vi "Creat_Traj_Config_Convert_V5_To_V_internal.vi"(11 "TrajCreateConfig V5":T5={"Write Config File Name"=path "", "Write Config File Comment"="", "WayPoints"=[], "TRAJECTORY_CONFIG_V4"={"MaxVelocity"=0.0, "Max Acceleration"=0.0, "StartVelocity"=0.0, "End Velocity"=0.0, "Reversed"=FALSE, "DiffDrKineConstntDefined"=FALSE, "CentAcellConstntDefined"=FALSE, "DiffDrVoltConstntDefined"=FALSE, "DIFF_DRIVE_KINE_CONSTRAINT"={"Max Speed (M/S)"=0.0, "DIFF_DRIVE_KINEMATICS"={"TrackWidth_Meters"=0.0}, "Max Accel (M/S2)"=99999.0}, "CENTRIPETAL_ACCEL_CONSTRAINT"={"Max Cent Accel"=0.0}, "SwerveDrKineConstntDefined"=FALSE, "SWERVE_DRIVE_KINE_CONSTRAINT"={"Max Speed (M/S)"=0.0, "SwerveKinematics"={"NumModules"=0, "InverseKinematics"=[], "ForwardKinematics"=[], "Modules"=[], "PrevCoR"={"X"=0.0, "Y"=0.0}, "SavedModuleStates"=[]}}, "DIFF_DRIVE_VOLTAGE_CONSTRAINT"={"Max Voltage"=0.0, "DIFF_DRIVE_KINEMATICS"={"TrackWidth_Meters"=0.0}, "SIMPLE_MOTOR_FF"={"Ks"=0.0, "Kv"=0.0, "Ka"=0.0, "KnInv"=0.0}}, "MECANUM_DRIVE_KINE_CONSTRAINT"={"Max Speed (M/S)"=0.0, "MECA_DRIVE_KINEMATICS"={"FrontLeft"={"X"=0.0, "Y"=0.0}, "FrontRight"={"X"=0.0, "Y"=0.0}, "RearLeft"={"X"=0.0, "Y"=0.0}, "RearRight"={"X"=0.0, "Y"=0.0}, "InverseKinematics"=[[0.0, 1.0, -1.0, 0.0], [0.0, 1.0, 1.0, 0.0], [0.0, 1.0, 1.0, 0.0], [0.0, 1.0, -1.0, 0.0]], "ForwardKinematics"=[[0.0, 1.0, -1.0, 0.0], [0.0, 1.0, 1.0, 0.0], [0.0, 1.0, 1.0, 0.0], [0.0, 1.0, -1.0, 0.0]], "PrevCoR"={"X"=0.0, "Y"=0.0}}}, "MecanumDrKineConstntDefined"=FALSE}, "IsCubic"=FALSE, "Units Selector"=enum."Inches", "UseWeights"=FALSE, "FieldName"="", "Rect Region Exists"=FALSE, "RectRegionBotLeft"={"X"=0.0, "Y"=0.0}, "RectRegionTopRight"={"X"=0.0, "Y"=0.0}, "Rect Region Max Speed"=0.0} {"RectRegionTopRight"."Y" format="%14.3f"; "RectRegionTopRight"."X" format="%14.3f"; "RectRegionBotLeft"."Y" format="%14.3f"; "RectRegionBotLeft"."X" format="%14.3f"; "WayPoints"."WEIGHT" format="%13.3f"; "WayPoints"."ANGLE" format="%13.3f"; "WayPoints"."Y" format="%13.3f"; "WayPoints"."X" format="%13.3f"; "TRAJECTORY_CONFIG_V4"."MECANUM_DRIVE_KINE_CONSTRAINT"."MECA_DRIVE_KINEMATICS"."PrevCoR"."Y" format="%14.3f"; "TRAJECTORY_CONFIG_V4"."MECANUM_DRIVE_KINE_CONSTRAINT"."MECA_DRIVE_KINEMATICS"."PrevCoR"."X" format="%14.3f"; "TRAJECTORY_CONFIG_V4"."MECANUM_DRIVE_KINE_CONSTRAINT"."MECA_DRIVE_KINEMATICS"."RearRight"."Y" format="%14.3f"; "TRAJECTORY_CONFIG_V4"."MECANUM_DRIVE_KINE_CONSTRAINT"."MECA_DRIVE_KINEMATICS"."RearRight"."X" format="%14.3f"; "TRAJECTORY_CONFIG_V4"."MECANUM_DRIVE_KINE_CONSTRAINT"."MECA_DRIVE_KINEMATICS"."RearLeft"."Y" format="%14.3f"; "TRAJECTORY_CONFIG_V4"."MECANUM_DRIVE_KINE_CONSTRAINT"."MECA_DRIVE_KINEMATICS"."RearLeft"."X" format="%14.3f"; "TRAJECTORY_CONFIG_V4"."MECANUM_DRIVE_KINE_CONSTRAINT"."MECA_DRIVE_KINEMATICS"."FrontRight"."Y" format="%14.3f"; "TRAJECTORY_CONFIG_V4"."MECANUM_DRIVE_KINE_CONSTRAINT"."MECA_DRIVE_KINEMATICS"."FrontRight"."X" format="%14.3f"; "TRAJECTORY_CONFIG_V4"."MECANUM_DRIVE_KINE_CONSTRAINT"."MECA_DRIVE_KINEMATICS"."FrontLeft"."Y" format="%14.3f"; "TRAJECTORY_CONFIG_V4"."MECANUM_DRIVE_KINE_CONSTRAINT"."MECA_DRIVE_KINEMATICS"."FrontLeft"."X" format="%14.3f"; "TRAJECTORY_CONFIG_V4"."MECANUM_DRIVE_KINE_CONSTRAINT"."Max Speed (M/S)" format="%20.4f"; "TRAJECTORY_CONFIG_V4"."DIFF_DRIVE_VOLTAGE_CONSTRAINT"."SIMPLE_MOTOR_FF"."KnInv" format="%13.4f"; "TRAJECTORY_CONFIG_V4"."DIFF_DRIVE_VOLTAGE_CONSTRAINT"."SIMPLE_MOTOR_FF"."Ka" format="%13.4f"; "TRAJECTORY_CONFIG_V4"."DIFF_DRIVE_VOLTAGE_CONSTRAINT"."SIMPLE_MOTOR_FF"."Kv" format="%13.4f"; "TRAJECTORY_CONFIG_V4"."DIFF_DRIVE_VOLTAGE_CONSTRAINT"."SIMPLE_MOTOR_FF"."Ks" format="%13.4f"; "TRAJECTORY_CONFIG_V4"."DIFF_DRIVE_VOLTAGE_CONSTRAINT"."DIFF_DRIVE_KINEMATICS"."TrackWidth_Meters" format="%20.4f"; "TRAJECTORY_CONFIG_V4"."DIFF_DRIVE_VOLTAGE_CONSTRAINT"."Max Voltage" format="%20.4f"; "TRAJECTORY_CONFIG_V4"."SWERVE_DRIVE_KINE_CONSTRAINT"."SwerveKinematics"."PrevCoR"."Y" format="%14.3f"; "TRAJECTORY_CONFIG_V4"."SWERVE_DRIVE_KINE_CONSTRAINT"."SwerveKinematics"."PrevCoR"."X" format="%14.3f"; "TRAJECTORY_CONFIG_V4"."SWERVE_DRIVE_KINE_CONSTRAINT"."SwerveKinematics"."Modules"."Y" format="%14.3f"; "TRAJECTORY_CONFIG_V4"."SWERVE_DRIVE_KINE_CONSTRAINT"."SwerveKinematics"."Modules"."X" format="%14.3f"; "TRAJECTORY_CONFIG_V4"."SWERVE_DRIVE_KINE_CONSTRAINT"."Max Speed (M/S)" format="%20.4f"; "TRAJECTORY_CONFIG_V4"."CENTRIPETAL_ACCEL_CONSTRAINT"."Max Cent Accel" format="%20.4f"; "TRAJECTORY_CONFIG_V4"."DIFF_DRIVE_KINE_CONSTRAINT"."Max Accel (M/S2)" format="%20.4f"; "TRAJECTORY_CONFIG_V4"."DIFF_DRIVE_KINE_CONSTRAINT"."DIFF_DRIVE_KINEMATICS"."TrackWidth_Meters" format="%20.4f"; "TRAJECTORY_CONFIG_V4"."DIFF_DRIVE_KINE_CONSTRAINT"."Max Speed (M/S)" format="%20.4f"; "TRAJECTORY_CONFIG_V4"."End Velocity" format="%20.4f"; "TRAJECTORY_CONFIG_V4"."StartVelocity" format="%20.4f"; "TRAJECTORY_CONFIG_V4"."Max Acceleration" format="%20.4f"; "TRAJECTORY_CONFIG_V4"."MaxVelocity" format="%20.4f"}) -> (3 "TrajCreateConfig V_Internal":T1 {"WayPoints"."WEIGHT" format="%13.3f"; "WayPoints"."ANGLE" format="%13.3f"; "WayPoints"."Y" format="%13.3f"; "WayPoints"."X" format="%13.3f"; "TRAJECTORY_CONFIG"."End Velocity" format="%20.4f"; "TRAJECTORY_CONFIG"."StartVelocity" format="%20.4f"; "TRAJECTORY_CONFIG"."Max Acceleration" format="%20.4f"; "TRAJECTORY_CONFIG"."MaxVelocity" format="%20.4f"})   [LabVIEW 2019]
uses:
  CreateTrajectoryTypeDef/TrajCreateConfig_V5.ctl
  <vilib>/Rock Robotics/WPI/ThirdParty/JAS_Junk/TrajLib/TypeDef/DISPLAY_WEIGHTED_WAYPOINT.ctl
  CreateTrajectoryTypeDef/TrajCreateTrajConfig_V4.ctl
  <vilib>/Rock Robotics/WPI/ThirdParty/JAS_Junk/TrajLib/TypeDef/TRAJ_CONSTRAINT_DIIF_DRIVE_KINEMATICS.ctl
  <vilib>/Rock Robotics/WPI/ThirdParty/JAS_Junk/TrajLib/TypeDef/DIFF_DRIVE_KINEMATICS.ctl
  <vilib>/Rock Robotics/WPI/ThirdParty/JAS_Junk/TrajLib/TypeDef/TRAJ_CONSTRAINT_CENTRIPETAL_ACCEL.ctl
  <vilib>/Rock Robotics/WPI/ThirdParty/JAS_Junk/TrajLib/TypeDef/TRAJ_CONSTRAINT_SWERVE_DRIVE_KINEMATICS.ctl
  <vilib>/Rock Robotics/WPI/ThirdParty/JAS_Junk/TrajLib/TypeDef/SWERVE_DRIVE_KINEMATICS.ctl
  <vilib>/Analysis/Matrix/Datatypes/RealMatrix.ctl
  <vilib>/Rock Robotics/WPI/ThirdParty/JAS_Junk/TrajLib/TypeDef/TRANSLATION2D.ctl
  <vilib>/Rock Robotics/WPI/ThirdParty/JAS_Junk/TrajLib/TypeDef/SWERVE_DRIVE_MODULE_STATE.ctl
  <vilib>/Rock Robotics/WPI/ThirdParty/JAS_Junk/TrajLib/TypeDef/ROTATION2D.ctl
  <vilib>/Rock Robotics/WPI/ThirdParty/JAS_Junk/TrajLib/TypeDef/TRAJ_CONSTRAINT_DIIF_DRIVE_VOLTAGE.ctl
  <vilib>/Rock Robotics/WPI/ThirdParty/JAS_Junk/TrajLib/TypeDef/SIMPLE_MOTOR_FF.ctl
  <vilib>/Rock Robotics/WPI/ThirdParty/JAS_Junk/TrajLib/TypeDef/TRAJ_CONSTRAINT_MECA_DRIVE_KINEMATICS.ctl
  <vilib>/Rock Robotics/WPI/ThirdParty/JAS_Junk/TrajLib/TypeDef/MECA_DRIVE_KINEMATICS.ctl
  CreateTrajectoryENUM/TrajCreateUnitsENUM.ctl
  CreateTrajectoryTypeDef/TrajCreateConfig__V_Internal.ctl
  <vilib>/Rock Robotics/WPI/ThirdParty/JAS_Junk/TrajLib/TypeDef/TRAJ_CONFIG.ctl
  <vilib>/Rock Robotics/WPI/ThirdParty/JAS_Junk/TrajLib/VI/TrajConstraint_GetType.vi
  <vilib>/Utility/Data Type/Get Type Information.vi
  <vilib>/Rock Robotics/WPI/ThirdParty/JAS_Junk/TrajLib/Trajectory_Library.lvlib
  <vilib>/Analysis/Matrix/NI_Matrix.lvlib
panel:
  # "ARRAY OF OTHER\nCONSTRAINTS \nGOES HERE.."
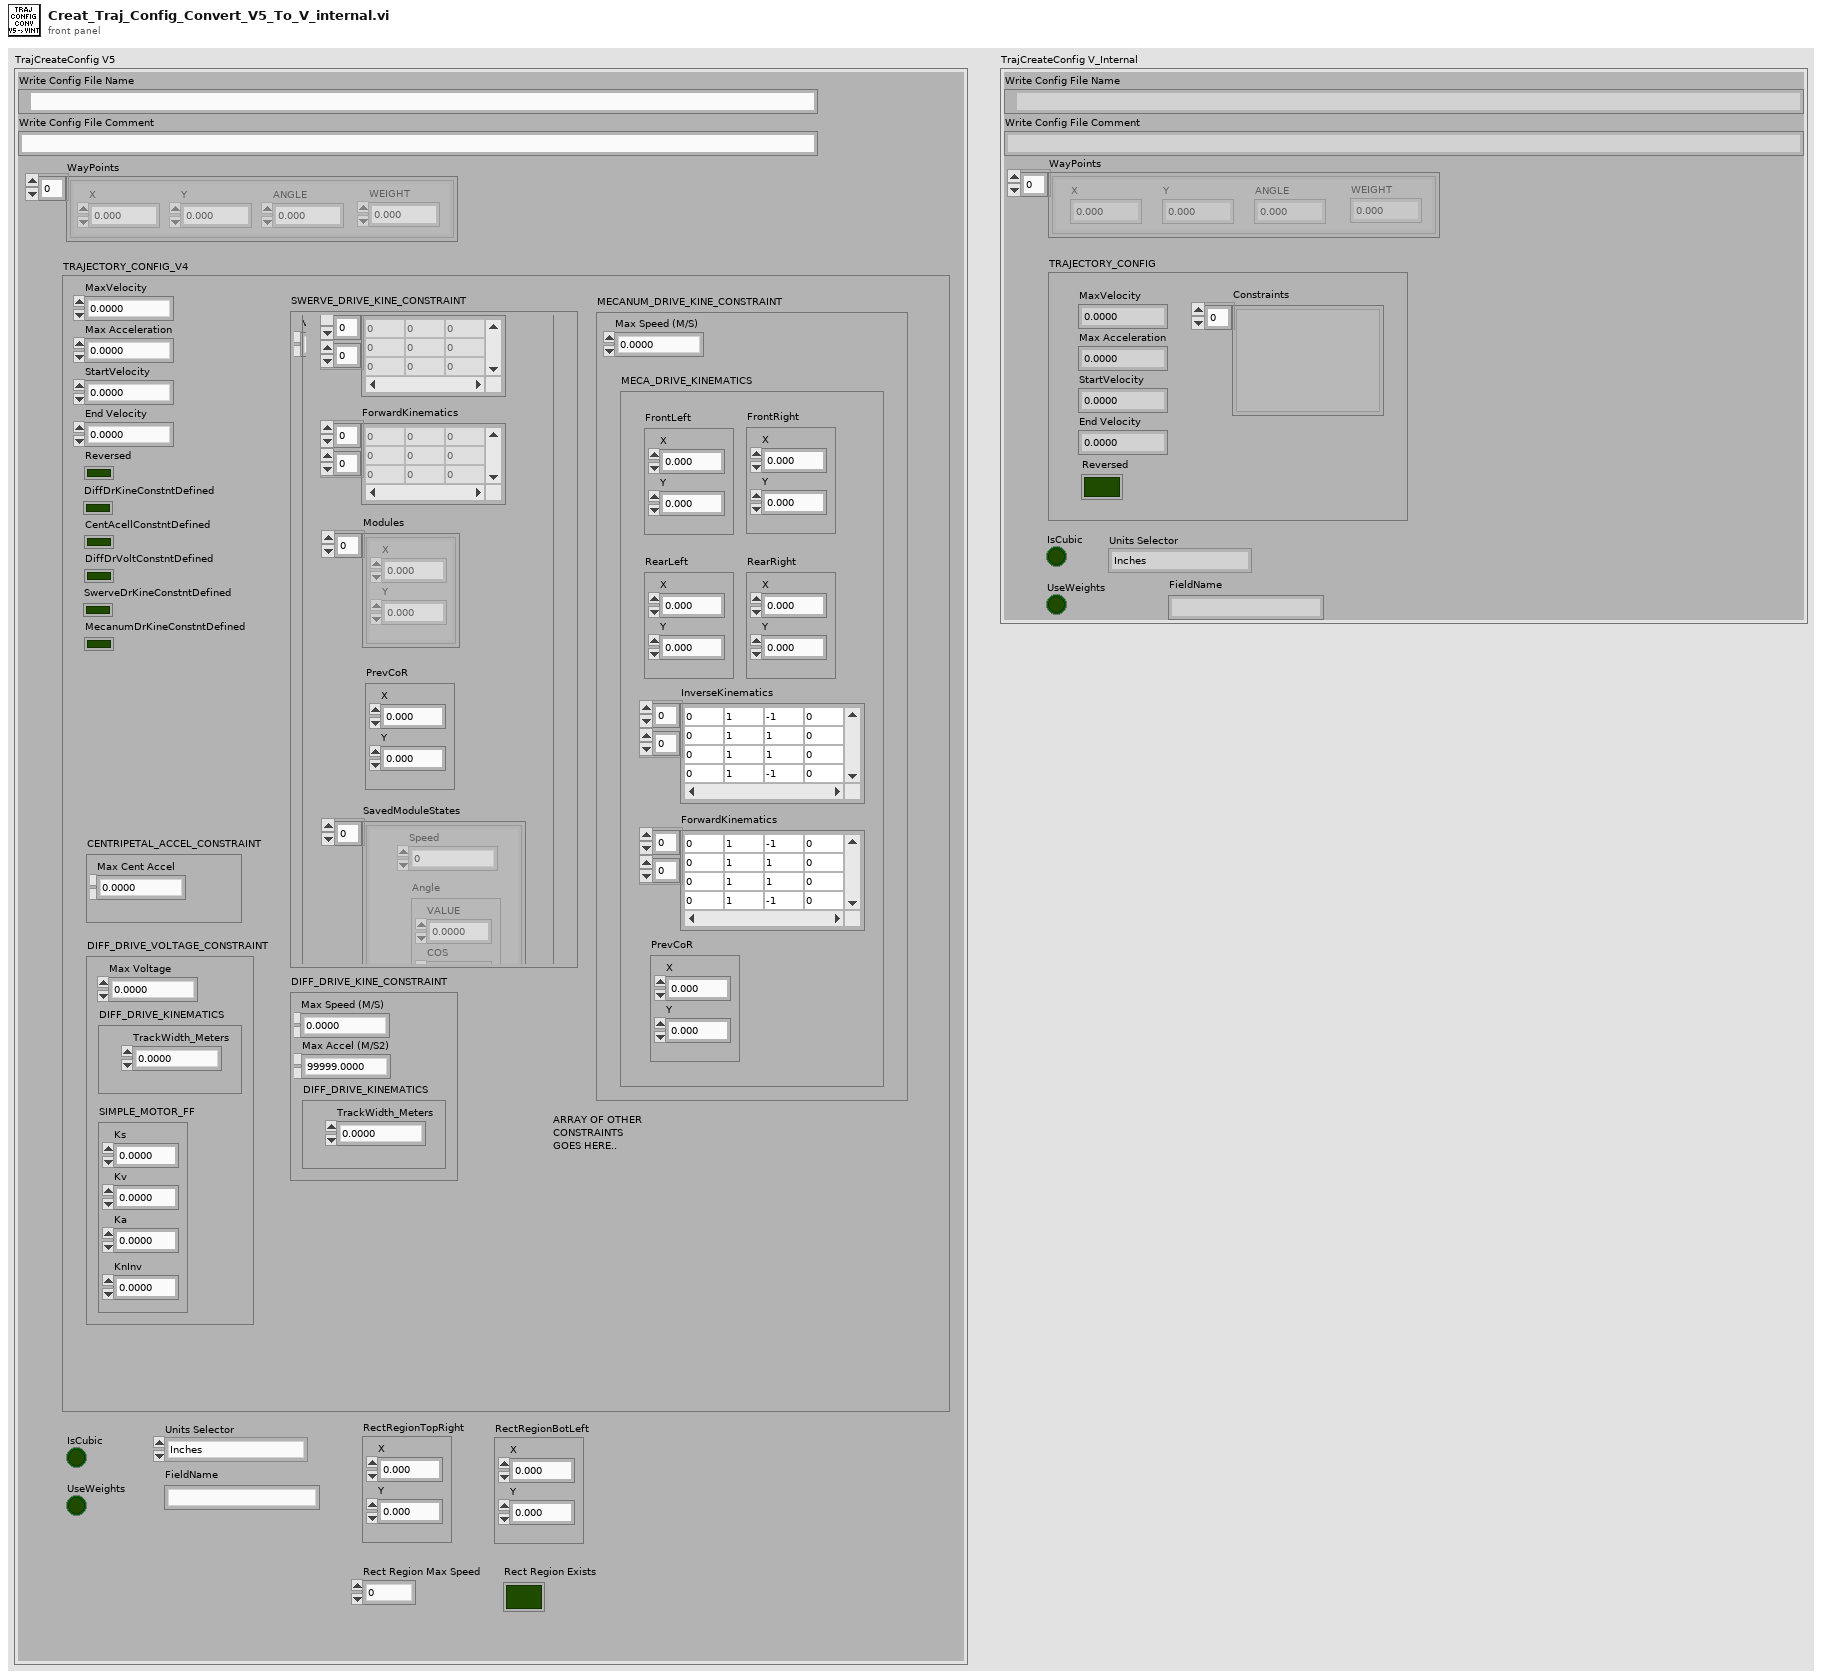
[diagram p1: front panel]
types:
  T1 = typedef "TrajCreateConfig__V_Internal.ctl" = cluster{"Write Config File Name":path, "Write Config File Comment":string, "WayPoints":T2[], "TRAJECTORY_CONFIG":T3, "IsCubic":bool, "Units Selector":T4, "UseWeights":bool, "FieldName":string}
  T2 = typedef "Trajectory_Library.lvlib/DISPLAY_WEIGHTED_WAYPOINT.ctl" = cluster{"X":dbl, "Y":dbl, "ANGLE":dbl, "WEIGHT":dbl}
  T3 = typedef "Trajectory_Library.lvlib/TRAJ_CONFIG.ctl" = cluster{"MaxVelocity":dbl, "Max Acceleration":dbl, "StartVelocity":dbl, "End Velocity":dbl, "Reversed":bool, "Constraints":variant[]}
  T4 = typedef "TrajCreateUnitsENUM.ctl" = enum16{"Inches", "Feet", "Centimeters", "Meters"}
  T5 = typedef "TrajCreateConfig_V5.ctl" = cluster{"Write Config File Name":path, "Write Config File Comment":string, "WayPoints":T2[], "TRAJECTORY_CONFIG_V4":T6, "IsCubic":bool, "Units Selector":T4, "UseWeights":bool, "FieldName":string, "Rect Region Exists":bool, "RectRegionBotLeft":T13, "RectRegionTopRight":T13, "Rect Region Max Speed":dbl}
  T6 = typedef "TrajCreateTrajConfig_V4.ctl" = cluster{"MaxVelocity":dbl, "Max Acceleration":dbl, "StartVelocity":dbl, "End Velocity":dbl, "Reversed":bool, "DiffDrKineConstntDefined":bool, "CentAcellConstntDefined":bool, "DiffDrVoltConstntDefined":bool, "DIFF_DRIVE_KINE_CONSTRAINT":T7, "CENTRIPETAL_ACCEL_CONSTRAINT":T9, "SwerveDrKineConstntDefined":bool, "SWERVE_DRIVE_KINE_CONSTRAINT":T10, "DIFF_DRIVE_VOLTAGE_CONSTRAINT":T16, "MECANUM_DRIVE_KINE_CONSTRAINT":T18, "MecanumDrKineConstntDefined":bool}
  T7 = typedef "Trajectory_Library.lvlib/TRAJ_CONSTRAINT_DIIF_DRIVE_KINEMATICS.ctl" = cluster{"Max Speed (M/S)":dbl, "DIFF_DRIVE_KINEMATICS":T8, "Max Accel (M/S2)":dbl}
  T8 = typedef "Trajectory_Library.lvlib/DIFF_DRIVE_KINEMATICS.ctl" = cluster{"TrackWidth_Meters":dbl}
  T9 = typedef "Trajectory_Library.lvlib/TRAJ_CONSTRAINT_CENTRIPETAL_ACCEL.ctl" = cluster{"Max Cent Accel":dbl}
  T10 = typedef "Trajectory_Library.lvlib/TRAJ_CONSTRAINT_SWERVE_DRIVE_KINEMATICS.ctl" = cluster{"Max Speed (M/S)":dbl, "SwerveKinematics":T11}
  T11 = typedef "Trajectory_Library.lvlib/SWERVE_DRIVE_KINEMATICS.ctl" = cluster{"NumModules":i32, "InverseKinematics":T12, "ForwardKinematics":T12, "Modules":T13[], "PrevCoR":T13, "SavedModuleStates":T14[]}
  T12 = typedef "NI_Matrix.lvlib/RealMatrix.ctl" = dbl[][]
  T13 = typedef "Trajectory_Library.lvlib/TRANSLATION2D.ctl" = cluster{"X":dbl, "Y":dbl}
  T14 = typedef "Trajectory_Library.lvlib/SWERVE_DRIVE_MODULE_STATE.ctl" = cluster{"Speed":dbl, "Angle":T15}
  T15 = typedef "Trajectory_Library.lvlib/ROTATION2D.ctl" = cluster{"VALUE":dbl, "COS":dbl, "SIN":dbl}
  T16 = typedef "Trajectory_Library.lvlib/TRAJ_CONSTRAINT_DIIF_DRIVE_VOLTAGE.ctl" = cluster{"Max Voltage":dbl, "DIFF_DRIVE_KINEMATICS":T8, "SIMPLE_MOTOR_FF":T17}
  T17 = typedef "Trajectory_Library.lvlib/SIMPLE_MOTOR_FF.ctl" = cluster{"Ks":dbl, "Kv":dbl, "Ka":dbl, "KnInv":dbl}
  T18 = typedef "Trajectory_Library.lvlib/TRAJ_CONSTRAINT_MECA_DRIVE_KINEMATICS.ctl" = cluster{"Max Speed (M/S)":dbl, "MECA_DRIVE_KINEMATICS":T19}
  T19 = typedef "Trajectory_Library.lvlib/MECA_DRIVE_KINEMATICS.ctl" = cluster{"FrontLeft":T13, "FrontRight":T13, "RearLeft":T13, "RearRight":T13, "InverseKinematics":T12, "ForwardKinematics":T12, "PrevCoR":T13}
  T20 = typedef "Trajectory_Library.lvlib/TRAJ_CONSTRAINT_MAX_VELOCITY.ctl" = cluster{"Max Velocity":dbl, "IM UNIQUE":bool}
  T21 = typedef "Trajectory_Library.lvlib/TRAJ_CONSTRAINT_RECT_REGION.ctl" = cluster{"BottomLeftPoint":T13, "TopRightPoint":T13, "Constraint":variant, "Constraint Type":T22}
  T22 = typedef "Trajectory_Library.lvlib/TRAJ_CONSTRAINT_TYPES_ENUM.ctl" = enum16{"UNDEFINED", "DIFF DRIVE KINEMATICS", "DIFF DRIVE VOLTAGE", "CENTRIPITAL ACCEL", "MECA DRIVE KINEMATICS", "SWERVE DRIVE KINEMATICS", "MAXIMUM VELOCITY", "ELLIPTICAL REGION", "RECTANGULAR REGION"}
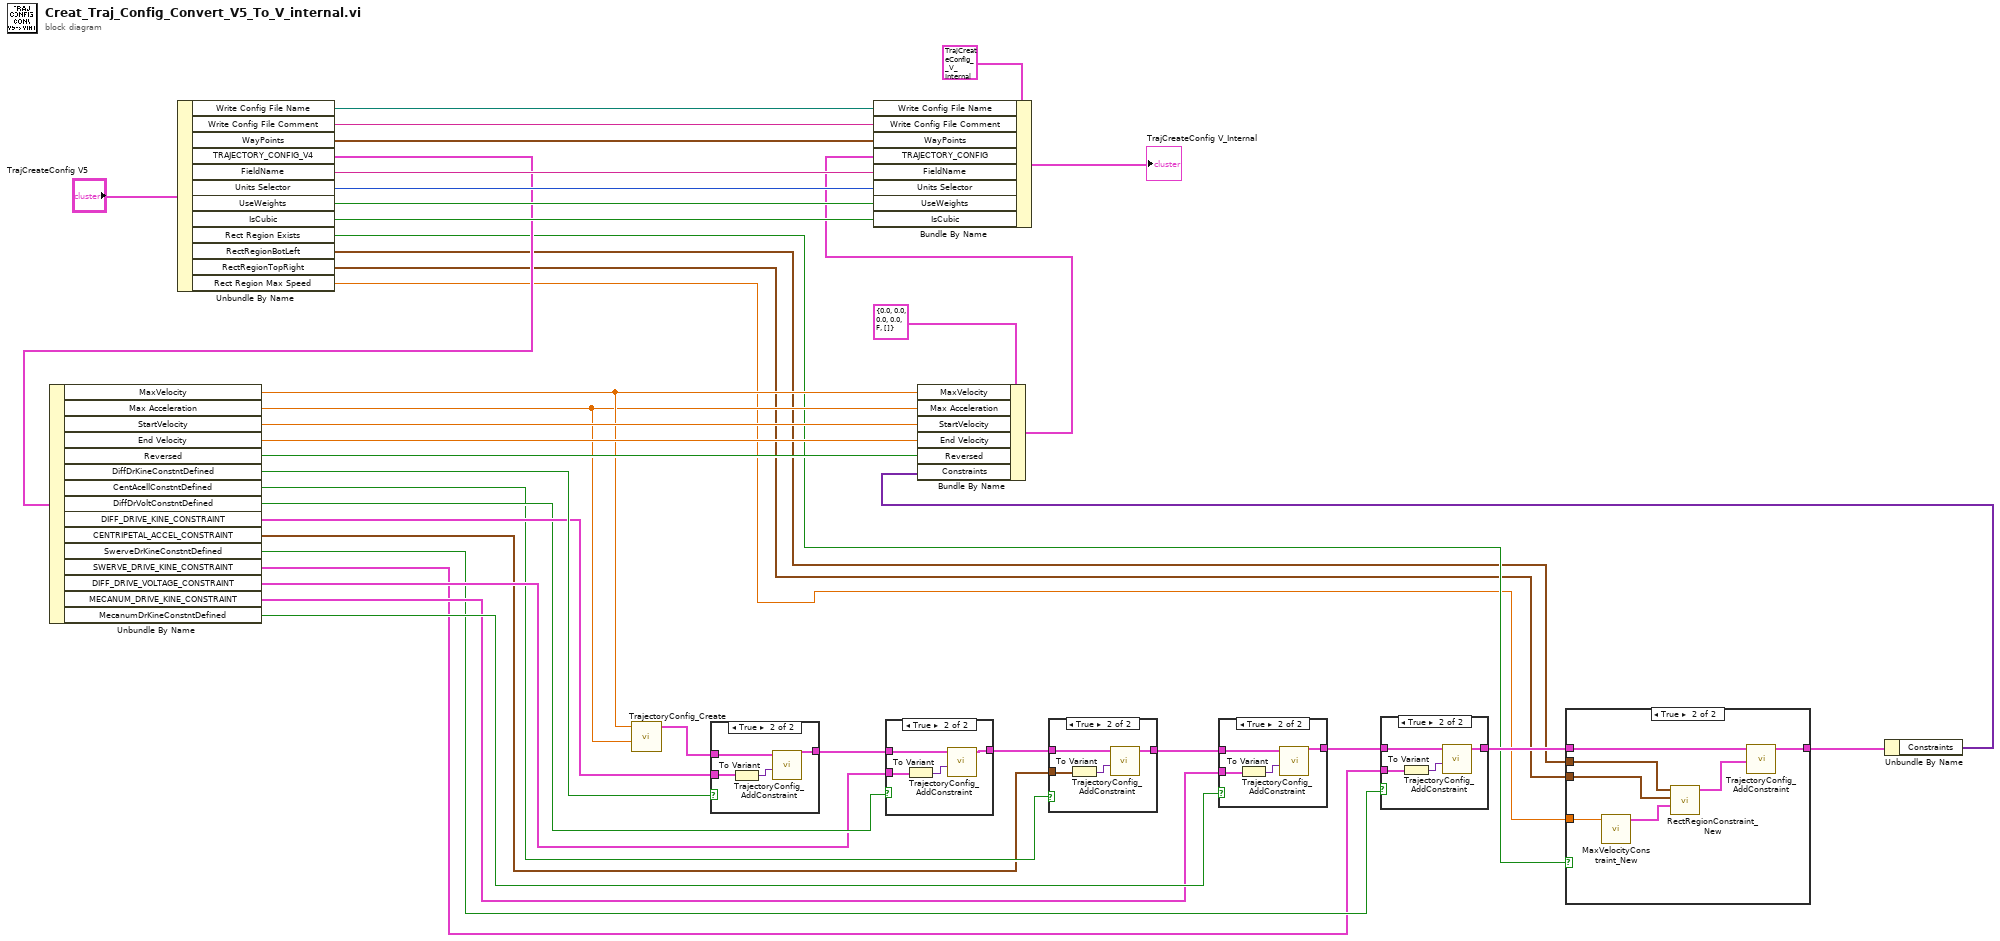
[diagram p0: block diagram]
diagram:
  n1 = Unbundle By Name("TrajCreateConfig V5") -> ("Write Config File Name"=w33:path, "Write Config File Comment"=w32:string, "WayPoints"=w31:T2[], "TRAJECTORY_CONFIG_V4"=w26:T6, "FieldName"=w30:string, "Units Selector"=w29:T4, "UseWeights"=w28:bool, "IsCubic"=w27:bool, "Rect Region Exists"=w6:bool, "RectRegionBotLeft"=w5:T13, "RectRegionTopRight"=w4:T13, "Rect Region Max Speed"=w1:dbl)
  n2 = Unbundle By Name(w26) -> ("MaxVelocity"=w21:dbl, "Max Acceleration"=w20:dbl, "StartVelocity"=w24:dbl, "End Velocity"=w23:dbl, "Reversed"=w22:bool, "DiffDrKineConstntDefined"=w18:bool, "CentAcellConstntDefined"=w14:bool, "DiffDrVoltConstntDefined"=w16:bool, "DIFF_DRIVE_KINE_CONSTRAINT"=w17:T7, "CENTRIPETAL_ACCEL_CONSTRAINT"=w13:T9, "SwerveDrKineConstntDefined"=w10:bool, "SWERVE_DRIVE_KINE_CONSTRAINT"=w9:T10, "DIFF_DRIVE_VOLTAGE_CONSTRAINT"=w15:T16, "MECANUM_DRIVE_KINE_CONSTRAINT"=w11:T18, "MecanumDrKineConstntDefined"=w12:bool)
  n3 = call <vilib>:"TrajectoryConfig_Create.vi"("MaxAcceleration"=w20, "MaxVelocity"=w21) -> ("TRAJECTORY_CONFIG"=w19:T3)  [unwired: 9 in]
  n4 = case shown="True" w18 {
    tunnel: w19 -> [w41 w44]
    tunnel: [w41 w43] -> w40
    tunnel: w17 -> [_ w42]
    frame False {
    }
    frame True {
      n5 = To Variant(anything=w42) -> (Variant=w45:variant)
      n6 = call <vilib>:"TrajectoryConfig_AddConstraint.vi"("Constraint"=w45, "inTRAJECTORY_CONFIG"=w44) -> ("outTRAJECTORY_CONFIG"=w43:T3)  [unwired: 9 in]
    }
  }
  n7 = case shown="True" w16 {
    tunnel: w40 -> [w46 w49]
    tunnel: [w46 w48] -> w39
    tunnel: w15 -> [_ w47]
    frame False {
    }
    frame True {
      n8 = To Variant(anything=w47) -> (Variant=w50:variant)
      n9 = call <vilib>:"TrajectoryConfig_AddConstraint.vi"("Constraint"=w50, "inTRAJECTORY_CONFIG"=w49) -> ("outTRAJECTORY_CONFIG"=w48:T3)  [unwired: 9 in]
    }
  }
  n10 = case shown="True" w14 {
    tunnel: w39 -> [w51 w54]
    tunnel: [w51 w53] -> w38
    tunnel: w13 -> [_ w52]
    frame False {
    }
    frame True {
      n11 = To Variant(anything=w52) -> (Variant=w55:variant)
      n12 = call <vilib>:"TrajectoryConfig_AddConstraint.vi"("Constraint"=w55, "inTRAJECTORY_CONFIG"=w54) -> ("outTRAJECTORY_CONFIG"=w53:T3)  [unwired: 9 in]
    }
  }
  n13 = case shown="True" w12 {
    tunnel: w38 -> [w56 w59]
    tunnel: [w56 w58] -> w37
    tunnel: w11 -> [_ w57]
    frame False {
    }
    frame True {
      n14 = To Variant(anything=w57) -> (Variant=w60:variant)
      n15 = call <vilib>:"TrajectoryConfig_AddConstraint.vi"("Constraint"=w60, "inTRAJECTORY_CONFIG"=w59) -> ("outTRAJECTORY_CONFIG"=w58:T3)  [unwired: 9 in]
    }
  }
  n16 = case shown="True" w10 {
    tunnel: w37 -> [w61 w64]
    tunnel: [w61 w63] -> w7
    tunnel: w9 -> [_ w62]
    frame False {
    }
    frame True {
      n17 = To Variant(anything=w62) -> (Variant=w65:variant)
      n18 = call <vilib>:"TrajectoryConfig_AddConstraint.vi"("Constraint"=w65, "inTRAJECTORY_CONFIG"=w64) -> ("outTRAJECTORY_CONFIG"=w63:T3)  [unwired: 9 in]
    }
  }
  n19 = case shown="True" w6 {
    tunnel: w7 -> [w66 w73]
    tunnel: w5 -> [_ w70]
    tunnel: w4 -> [_ w69]
    tunnel: [w66 w72] -> w3
    tunnel: w1 -> [_ w71]
    frame False {
    }
    frame True {
      n20 = call <vilib>:"MaxVelocityConstraint_New.vi"("Maximum Velocity"=w71) -> ("MAX_VELOCITY_CONSTRAINT"=w68:T20)  [unwired: 10 in]
      n21 = call <vilib>:"RectRegionConstraint_New.vi"("Constraint Data Cluster"=w68, "TopRightPoint"=w69, "BottomLeftPoint"=w70) -> ("RECT_REGION_CONSTRAINT"=w67:T21)  [unwired: 8 in]
      n22 = call <vilib>:"TrajectoryConfig_AddConstraint.vi"("Constraint"=w67, "inTRAJECTORY_CONFIG"=w73) -> ("outTRAJECTORY_CONFIG"=w72:T3)  [unwired: 9 in]
    }
  }
  n23 = Unbundle By Name(w3) -> ("Constraints"=w2:variant[])
  n24 = Bundle By Name(cluster=T3 {"MaxVelocity"=0.0, "Max Acceleration"=0.0, "StartVelocity"=0.0, "End Velocity"=0.0, "Reversed"=FALSE, "Constraints"=[]} ("TRAJECTORY_CONFIG"), "MaxVelocity"=w21, "Max Acceleration"=w20, "StartVelocity"=w24, "End Velocity"=w23, "Reversed"=w22, "Constraints"=w2) -> (w8:T3)
  n25 = Bundle By Name(cluster=T1 {"Write Config File Name"=path "", "Write Config File Comment"="", "WayPoints"=[], "TRAJECTORY_CONFIG"={"MaxVelocity"=0.0, "Max Acceleration"=0.0, "StartVelocity"=0.0, "End Velocity"=0.0, "Reversed"=FALSE, "Constraints"=[]}, "IsCubic"=FALSE, "Units Selector"=enum."Inches", "UseWeights"=FALSE, "FieldName"=""} ("TrajCreateConfig"), "Write Config File Name"=w33, "Write Config File Comment"=w32, "WayPoints"=w31, "TRAJECTORY_CONFIG"=w8, "FieldName"=w30, "Units Selector"=w29, "UseWeights"=w28, "IsCubic"=w27) -> (→"TrajCreateConfig V_Internal":T1)
